vi "Create_New_Build.vi"(6 "buildSpecName":string, 7 "Programmatic? (false)":bool, 8 "error in (no error)":errorcluster, 9 "buildObject":T1, 10 "Destination Path":path, 11 "AB_DepPackedLibrary in":refnum<class "AB_DepPackedLibrary.lvclass">) -> (0 "error out":errorcluster, 3 "AB_DepPackedLibrary out":refnum<class "AB_DepPackedLibrary.lvclass">)   [LabVIEW 2020, in "AB_DepPackedLibrary.lvclass"]
uses:
  <vilib>/AppBuilder/AB_Classes/DepPackedLib/AB_DepPackedLibrary.lvclass
  e:/builds/penguin/labview/branches/2020/dev/dist/vi.lib/AppBuilder/AB_Classes/Build/AB_Build.lvclass
  <resource>/Framework/Providers/API/ItemRef.ctl
  <vilib>/AppBuilder/AB_Classes/PackedLib/AB_PackedLibrary.lvclass
  <vilib>/AppBuilder/AB_Classes/Deployment/AB_Deployment.lvlib
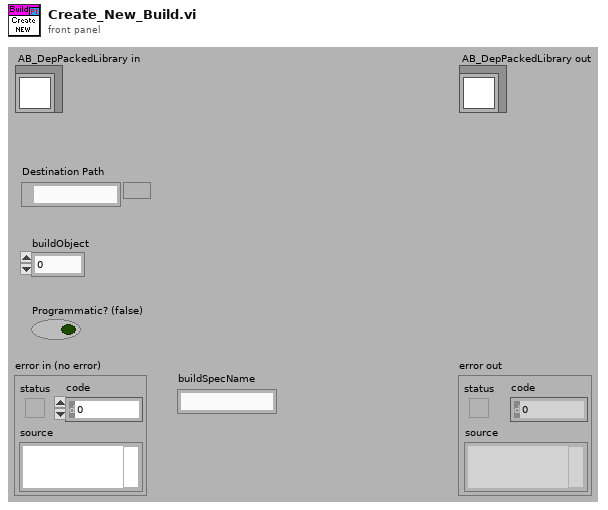
[diagram p1: front panel]
types:
  T1 = typedef "ItemRef.ctl" = u64
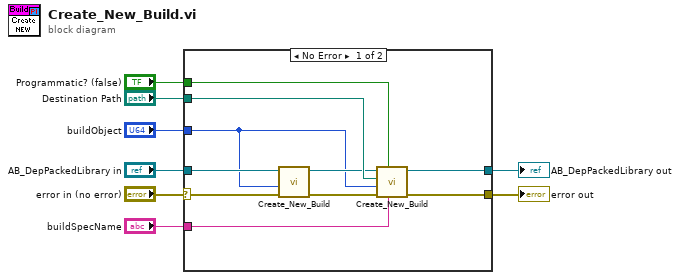
[diagram p0: block diagram]
diagram:
  n1 = case shown="No Error" "error in (no error)" {
    selector: "error in (no error)" -> [w11 w19]
    tunnel: "buildSpecName" -> [w18 _]
    tunnel: "Programmatic? (false)" -> [w17 _]
    tunnel: "buildObject" -> [w9 _]
    tunnel: "Destination Path" -> [w16 _]
    tunnel: "AB_DepPackedLibrary in" -> [w13 w20]
    tunnel: [w15 w19] -> w3
    tunnel: [w14 w20] -> w2
    frame No Error {
      n2 = call <vilib>:"Create_New_Build.vi"("error in (no error)"=w11, "buildObject"=w9, "Build in"=w13) -> ("error out"=w10:errorcluster, "Build out"=w12:refnum<class "AB_DepPackedLibrary.lvclass">)  [unwired: 7 in]
      n3 = call-parent <vilib>:"Create_New_Build.vi"("buildSpecName"=w18, "Programmatic? (false)"=w17, "error in (no error)"=w10, "buildObject"=w9, "Destination Path"=w16, "AB_PackedLibrary in"=w12) -> ("error out"=w15:errorcluster, "AB_PackedLibrary out"=w14:refnum<class "AB_DepPackedLibrary.lvclass">)  [unwired: 4 in]
    }
    frame Error {
    }
  }
  "error out" <- w3
  "AB_DepPackedLibrary out" <- w2
